vi "(SubVI) Initiate Queue.vi"() -> (3 "Cluster":T2)   [LabVIEW 2014]
uses:
  <vilib>/vision/Image Controls.llb/IMAQ Image.ctl
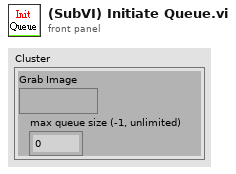
[diagram p1: front panel]
types:
  T1 = typedef "IMAQ Image.ctl" = refnum<image>
  T2 = cluster{"Grab Image":T1, "max queue size (-1, unlimited)":u32}
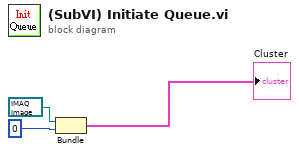
[diagram p0: block diagram]
diagram:
  n1 = Bundle("Grab Image"=T1 refnum, "max queue size (-1, unlimited)"=u32 0) -> (→"Cluster":T2)  [unwired: 1 in]
